vi "SCMP - print screen.vi"(7 "mode (save)":enum16{"Init", "Save"}(ring)=enum."Save", 8 "error in (no error)":errorcluster, 10 "image data":T1, 11 "FITS Header in":T2={"Wavelength (nm)"=530.15, "Exposure (s)"=0.05, "Tuning Delay (ms)"=200.0, "Beam Type (-1/1)"=1.0, "Tuning Voltages"=[1.111, 2.222, 3.333, 4.444], "Observer"="observer", "Light Shapping Diffuser"=enum."In Beam", "Comment"="", "Data Type"=enum."LIVE", "Mod Cycles"=1, "SCD Calibration Optics"=enum."1 - Polarizer @0, I+Q", "SCD Emission Line Filter"=enum."1-557.6nm", "Cookbook"="", "COMP-S Calibration Wheel"=enum."Dark", "COMP-S Andover Filter Wheel"=enum."530.3nm/HWB 0.34nm (Fe XIV)", "FOV Rotation (deg)"=66.0, "Objective Lens Position (mm)"=0.0, "Occulter size"=0.0, "Time End"=timestamp(3382374145.421875 s since 1904-01-01), "Acc Exposure (s)"=0.0, "Time Stamp Array"=[], "Camera Serial Number"=[], "Camera Temp"=[], "Camera PI (mm)"=[0.0, 0.0, 0.0], "Time Start"=timestamp(3382374145.421875 s since 1904-01-01), "Peripherals"={"ILX controler"=FALSE, "Zone temperatures"=FALSE, "Andor"=FALSE, "Andor 2"=FALSE, "PI Stages"=FALSE, "AISAS mechanisms"=FALSE, "AISAS Mech.lvclass"=refnum, "Zone temp ref"=variant, "FWs"=FALSE}, "FITS paths"=[], "Cameras"=enum."Andor", "load preset cbk"=FALSE, "periodic check count"=0, "COMP-S Calibration Wheel 2"=enum."Dark", "Calib"=enum."Dark", "Abso Aperture"=66.0, "Nominal Aperture"=66.0, "Pointer IP"="127.0.0.1"} {"Nominal Aperture" format="%.1f"; "Abso Aperture" format="%.1f"; "Camera PI (mm)" format="%_3g"; "Acc Exposure (s)" format="%^.3g"; "Occulter size" format="%.2f"; "Objective Lens Position (mm)" min=70.0 max=152.0 format="%.2f"; "FOV Rotation (deg)" format="%.1f"; "Exposure (s)" format="%^.3g"; "Wavelength (nm)" format="%_6g"}) -> (0 "error out":errorcluster, 3 "FITS Header out":T2={"Wavelength (nm)"=0.0, "Exposure (s)"=0.0, "Tuning Delay (ms)"=0.0, "Beam Type (-1/1)"=0.0, "Tuning Voltages"=[], "Observer"="", "Light Shapping Diffuser"=enum."Out of Beam", "Comment"="", "Data Type"=enum."LIVE", "Mod Cycles"=0, "SCD Calibration Optics"=enum."1 - Polarizer @0, I+Q", "SCD Emission Line Filter"=enum."1-557.6nm", "Cookbook"="", "COMP-S Calibration Wheel"=enum."Dark", "COMP-S Andover Filter Wheel"=enum."530.3nm/HWB 0.34nm (Fe XIV)", "FOV Rotation (deg)"=0.0, "Objective Lens Position (mm)"=0.0, "Occulter size"=0.0, "Time End"=timestamp(0 s since 1904-01-01), "Acc Exposure (s)"=0.0, "Time Stamp Array"=[], "Camera Serial Number"=[], "Camera Temp"=[], "Camera PI (mm)"=[], "Time Start"=timestamp(0 s since 1904-01-01), "Peripherals"={"ILX controler"=FALSE, "Zone temperatures"=FALSE, "Andor"=FALSE, "Andor 2"=FALSE, "PI Stages"=FALSE, "AISAS mechanisms"=FALSE, "AISAS Mech.lvclass"=refnum, "Zone temp ref"=variant, "FWs"=FALSE}, "FITS paths"=[], "Cameras"=enum."Andor", "load preset cbk"=FALSE, "periodic check count"=0, "COMP-S Calibration Wheel 2"=enum."Dark", "Calib"=enum."Dark", "Abso Aperture"=66.0, "Nominal Aperture"=66.0, "Pointer IP"="127.0.0.1"} {"Nominal Aperture" format="%.1f"; "Abso Aperture" format="%.1f"; "Camera PI (mm)" format="%_3g"; "Acc Exposure (s)" format="%^.3g"; "Occulter size" format="%.2f"; "Objective Lens Position (mm)" min=70.0 max=152.0 format="%.2f"; "FOV Rotation (deg)" format="%.1f"; "Exposure (s)" format="%^.3g"; "Wavelength (nm)" format="%_6g"})   [LabVIEW 2014]
uses:
  Controls/SCD - FITS Cluster.ctl
  AISAS/Mech/AISAS Mech.lvclass
  AISAS/Controls/Diffuser.ctl
  Controls/FITS Data type.ctl
  Controls/SCD - Calibration Optics Filter Wheel.ctl
  Controls/SCD - EDT - Emission Line Filter Wheel.ctl
  Controls/CoMP-S Controls/Polarization Optics Filter Wheel.ctl
  Controls/CoMP-S Controls/Emission Line Filter Wheel.ctl
  AISAS/Controls/focus.ctl
  Controls/peripherals.ctl
  Controls/Cameras select.ctl
  <vilib>/picture/picture.llb/imagedata.ctl
  Controls/Globals.vi
panel:
  out "printsreen path":path
  out "file name":string
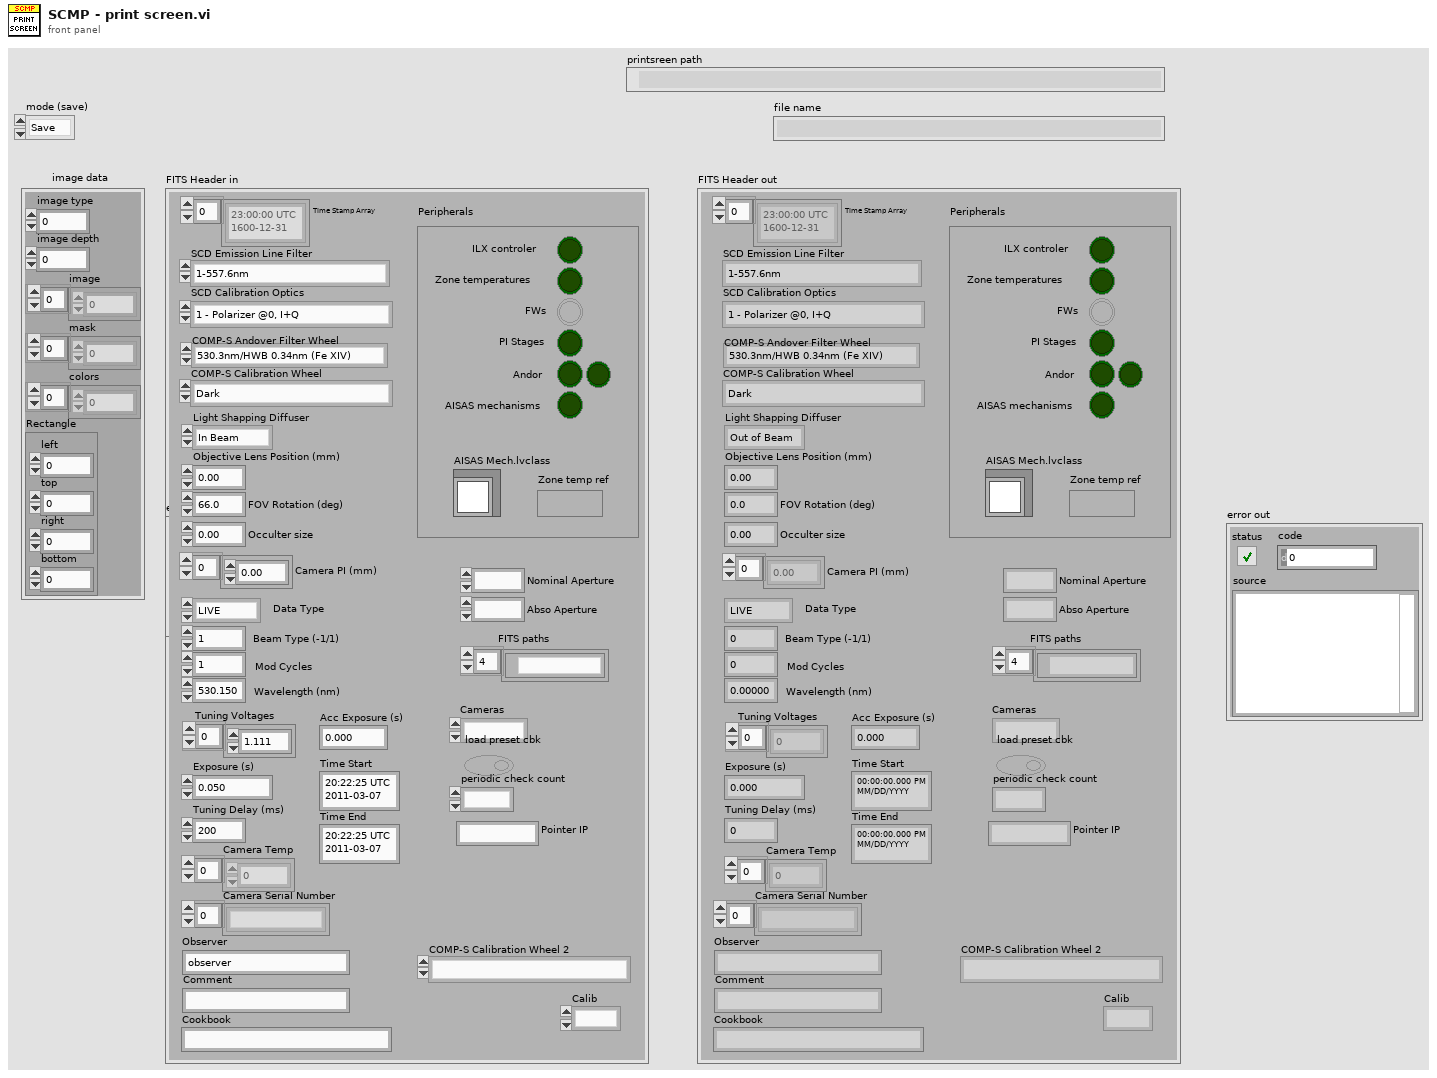
[diagram p1: front panel]
types:
  T1 = typedef "imagedata.ctl" = cluster{"image type":i32, "image depth":i32, "image":u8[], "mask":u8[], "colors":u32[], "Rectangle":cluster{"left":i16, "top":i16, "right":i16, "bottom":i16}}
  T2 = typedef "SCD - FITS Cluster.ctl" = cluster{"Wavelength (nm)":dbl, "Exposure (s)":dbl, "Tuning Delay (ms)":dbl, "Beam Type (-1/1)":dbl, "Tuning Voltages":dbl[], "Observer":string, "Light Shapping Diffuser":T3, "Comment":string, "Data Type":T4, "Mod Cycles":u16, "SCD Calibration Optics":T5, "SCD Emission Line Filter":T6, "Cookbook":string, "COMP-S Calibration Wheel":T7, "COMP-S Andover Filter Wheel":T8, "FOV Rotation (deg)":dbl, "Objective Lens Position (mm)":T9, "Occulter size":dbl, "Time End":timestamp, "Acc Exposure (s)":dbl, "Time Stamp Array":timestamp[], "Camera Serial Number":string[], "Camera Temp":dbl[], "Camera PI (mm)":dbl[], "Time Start":timestamp, "Peripherals":T10, "FITS paths":path[], "Cameras":T11, "load preset cbk":bool, "periodic check count":i32, "COMP-S Calibration Wheel 2":T7, "Calib":enum16{"Dark", "Flat"}, "Abso Aperture":dbl, "Nominal Aperture":dbl, "Pointer IP":string}
  T3 = typedef "Diffuser.ctl" = enum16{"Out of Beam", "In Beam"}
  T4 = typedef "FITS Data type.ctl" = enum16{"LIVE", "DARK", "FLAT", "CALI", "OBSE", "ABSO", "AURE", "TARG", "OBJE", "HOLE", "OREX", "THRO", "CHIP"}
  T5 = typedef "SCD - Calibration Optics Filter Wheel.ctl" = enum16{"1 - Polarizer @0, I+Q", "2 - Polarizer @90, I-Q", "3 - Polarizer @45, I+U", "4 - Polarizer @135, I-U", "5 - Polarizer @0, Retarder @45, I+V", "6 - Polarizer @0, Retarder @135, I-V", "7 - Dark", "8 - Clear", "9 - N/A"}
  T6 = typedef "SCD - EDT - Emission Line Filter Wheel.ctl" = enum16{"1-557.6nm", "2-587.6nm", "3-589.6nm", "4-630.2nm", "5-656.4nm", "6-849.8nm", "7-854.2nm", "8-866.2nm", "9-1083.0nm"}
  T7 = typedef "Polarization Optics Filter Wheel.ctl" = enum16{"Dark", "Clear", "Exchange Lens", "Polarizer @0, I+Q", "Polarizer @90, I-Q", "Polarizer @45, I+U", "Polarizer @135, I-U", "Polarizer @0, Retarder @45, I+V", "Polarizer @0, Retarder @135, I-V"}
  T8 = typedef "Emission Line Filter Wheel.ctl" = enum16{"530.3nm/HWB 0.34nm (Fe XIV)", "587.6nm/HBW 0.44nm (He I D3)", "637.5nm/HBW 0.53nm (Fe X)", "656.3nm/HBW 0.57nm (H-Alpha)", "789.2nm/HBW 0.85nm (Fe XI)", "854.2nm/HBW 1.01nm (Ca I)", "1074.7nm/HBW 2.34nm (Fe XIII)", "1079.8nm/HBW 1.64nm (Fe XIII)", "1083.0nm/HBW 1.66nm (He I)"}
  T9 = typedef "focus.ctl" = dbl
  T10 = typedef "peripherals.ctl" = cluster{"ILX controler":bool, "Zone temperatures":bool, "Andor":bool, "Andor 2":bool, "PI Stages":bool, "AISAS mechanisms":bool, "AISAS Mech.lvclass":refnum<class "AISAS Mech.lvclass">, "Zone temp ref":variant, "FWs":bool}
  T11 = typedef "Cameras select.ctl" = enum16{"Andor", "GDR"}
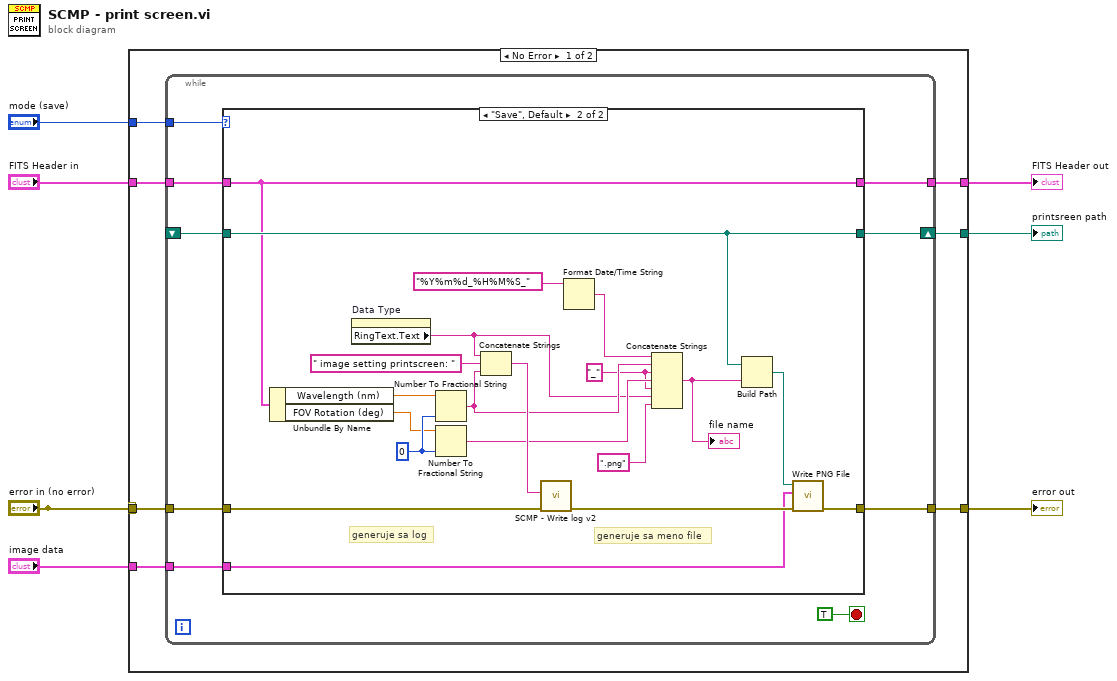
[diagram p0: block diagram]
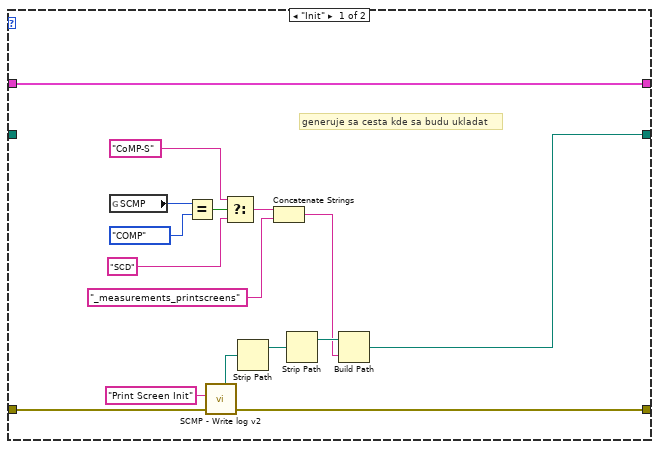
[diagram p2: hidden frame]
diagram:
  n1 = case shown="No Error" "error in (no error)" {
    selector: "error in (no error)" -> [w13 w61]
    tunnel: "error in (no error)" -> [_ _]
    tunnel: [w10 w60] -> w7
    tunnel: "FITS Header in" -> [w12 w60]
    tunnel: [w11 w61] -> w5
    tunnel: "mode (save)" -> [w14 _]
    tunnel: "image data" -> [w9 _]
    tunnel: [w8 _] -> w1
    frame No Error {
      n2 = while {
        tunnel: w14 -> [w22]
        tunnel: w13 -> [w21]
        shift-right: [w20] -> w8
        shift-left: _ -> [w19]
        tunnel: w12 -> [w18]
        tunnel: [w17] -> w11
        tunnel: [w16] -> w10
        tunnel: w9 -> [w15]
        stop <- TRUE stop-if-true
        n3 = case shown="\"Save\", Default" w22 {
          tunnel: w21 -> [w39 w59]
          tunnel: [w34 w51] -> w20
          tunnel: w19 -> [_ w51]
          tunnel: w18 -> [w24 w46]
          tunnel: [w25 w48] -> w17
          tunnel: [w24 w46] -> w16
          tunnel: w15 -> [_ w45]
          frame "Init" {
            # "generuje sa cesta kde sa budu ukladat"
            n4 = global read "Globals.vi" "SCMP"() -> (w33:enum16{"COMP", "SCD"})
            n5 = Equal?(x=w33, y=enum16{"COMP", "SCD"}."COMP") -> (x = y?=w31:bool)
            n6 = call "SCMP - Write log v2.vi"("Error to log"=w39, "data"="Print Screen Init") -> ("error out"=w25:errorcluster, "Today's SCMP Log File"=w37:path)  [unwired: 7 in, 1 out]
            n7 = Select(t="CoMP-S" ("name or relative path"), s=w31, f="SCD" ("name or relative path")) -> (s? t:f=w28:string)
            n8 = Strip Path(path=w37) -> (stripped path=w36:path)  [unwired: 1 out]
            n9 = Concatenate Strings(w28, "_measurements_printscreens" ("name or relative path")) -> (w26:string)
            n10 = Strip Path(path=w36) -> (stripped path=w35:path)  [unwired: 1 out]
            n11 = Build Path(base path=w35, name or relative path=w26) -> (appended path=w34:path)
          }
          frame "Save", Default {
            w42 = "_" ("string")
            w54 = i16 0 ("precision (6)")
            # "generuje sa meno file"
            # "generuje sa log"
            n12 = Unbundle By Name(w46) -> ("Wavelength (nm)"=w56:dbl, "FOV Rotation (deg)"=w53:dbl)
            n13 = property on="Data Type" class="Enum (strict)"() -> ("RingText.Text"=w41:string)  [unwired: 2 in, 2 out]
            n14 = Number To Fractional String(number=w56, precision (6)=w54) -> (F-format string=w55:string)  [unwired: 2 in]
            n15 = Number To Fractional String(number=w53, precision (6)=w54) -> (F-format string=w52:string)  [unwired: 2 in]
            n16 = Concatenate Strings(w41, " image setting printscreen: " ("data"), w55) -> (w57:string)
            n17 = call "SCMP - Write log v2.vi"("Error to log"=w59, "data"=w57) -> ("error out"=w49:errorcluster)  [unwired: 7 in, 2 out]
            n18 = Format Date/Time String(time format string (%c)="%Y%m%d_%H%M%S_") -> (date/time string=w43:string)  [unwired: 2 in]
            n19 = Concatenate Strings(w43, w55, w42, w52, w42, w41, ".png" ("time format string (%c)")) -> (w50:string)
            "file name" <- w50
            n20 = Build Path(base path=w51, name or relative path=w50) -> (appended path=w47:path)
            n21 = call <vilib>:"Write PNG File.vi"("error in (no error)"=w49, "image data"=w45, "path to PNG file"=w47) -> ("error out"=w48:errorcluster)  [unwired: 7 in, 1 out]
          }
        }
      }
    }
    frame Error {
    }
  }
  "FITS Header out" <- w7
  "error out" <- w5
  "printsreen path" <- w1
